vi "485 comm Main Page.vi"(8 "error in (no error)":errorcluster, 11 "Node Ptr":T3 format="%.0x") -> (0 "error out":errorcluster)   [LabVIEW 2015, in "485 comm Custom Device.lvlib"]
uses:
  485 comm Custom Device.lvlib
  <vilib>/NI Veristand/Custom Device API/Custom Device API.lvlib
  <vilib>/NI Veristand/Custom Device API/Set Item Property (U32).vi
  Serial - Settings.ctl
  <vilib>/NI Veristand/Custom Device API/Set Item Property (Boolean).vi
  <vilib>/NI Veristand/Custom Device API/Set Item Property (Variant).vi
  <vilib>/NI Veristand/Custom Device API/Get Item Property (Boolean).vi
  <vilib>/NI Veristand/Custom Device API/Set Item Property (String).vi
  <vilib>/NI Veristand/Custom Device API/Set Item Property (U16).vi
  <vilib>/NI Veristand/Custom Device API/Get Item Property (U32).vi
  <vilib>/NI Veristand/Custom Device API/Get Item Property (Variant).vi
  <vilib>/NI Veristand/Custom Device API/Get Item Property (String).vi
  <vilib>/NI Veristand/Custom Device API/Get Item Property (U16).vi
  <vilib>/NI Veristand/Custom Device API/Custom Device Channel Type.ctl
  <vilib>/NI Veristand/Custom Device API/Custom Device Channel.ctl
  <vilib>/NI Veristand/Custom Device API/Custom Device Item Ref.ctl
panel:
  in  "add output channel":bool
  in  "add input channel":bool
  in  "Reuse Old Data?":bool
  in  "Period (ms)":u32=1000
  in  "Timeout (s)":u32=10
  in  "RS-485 Transceiver Mode":T1(ring)
  in  "VISA resource":refnum<visa-resource-name>="COM3"
  in  "Serial Settings":T2={"baud rate"=9600, "data bits"=8, "parity"=enum."None", "stop bits"=10, "flow control"=0} {"flow control" items=["None"=0, "XON/XOFF"=1, "RTS/CTS"=2, "DTR/DSR"=4]; "stop bits" items=["1.0"=10, "1.5"=15, "2.0"=20]; "data bits" min=5 max=8 step=1; "baud rate" items=["75"=75, "110"=110, "134"=134, "150"=150, "300"=300, "600"=600, "1200"=1200, "1800"=1800, "2400"=2400, "4800"=4800, "7200"=7200, "9600"=9600, "14400"=14400, "19200"=19200, "28800"=28800, "38400"=38400, "56000"=56000, "57600"=57600, "115200"=115200, "128000"=128000, "230400"=230400, "921600"=921600]}
  in  "Header":cluster{"Section Name":string}={"Section Name"="Custom Device Item Settings"}
  in  "Description":string
  in  "Name":string
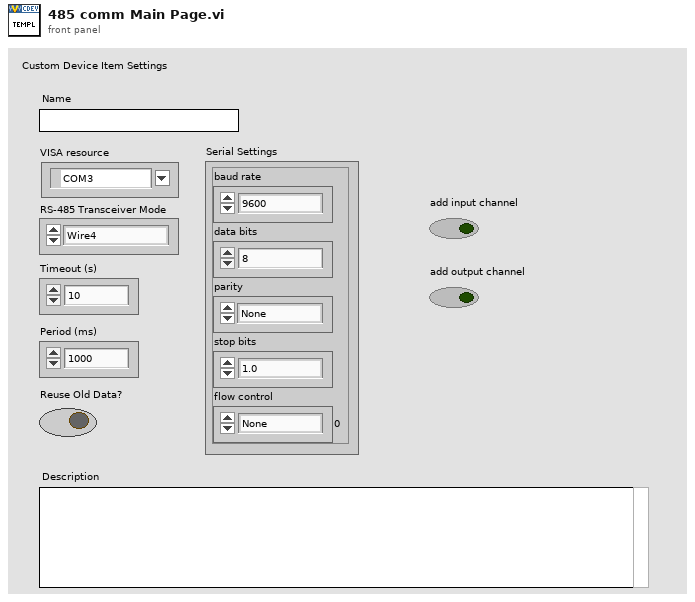
[diagram p1: front panel]
types:
  T1 = enum16{"Wire4", "Wire2-EchoDTR", "Wire2-CtrlDTR", "Wire2-Auto"}
  T2 = typedef "485 comm Custom Device.lvlib/Serial - Settings.ctl" = cluster{"baud rate":u32, "data bits":u16, "parity":enum16{"None", "Odd", "Even", "Mark", "Space"}, "stop bits":u16, "flow control":u16}
  T3 = typedef "Custom Device API.lvlib/Custom Device Item Ref.ctl" = u64
  T4 = typedef "Custom Device API.lvlib/Custom Device Item Info.ctl" = cluster{"Name":string, "Is Channel":bool, "GUID":string, "Is Waveform":bool}
  T5 = typedef "Custom Device API.lvlib/Custom Device Channel.ctl" = cluster{"Type":T6, "Units":string, "Default Value":dbl, "Faultable":bool, "Scalable":bool}
  T6 = typedef "Custom Device API.lvlib/Custom Device Channel Type.ctl" = enum16{"Input", "Output"}
  T7 = typedef "Custom Device API.lvlib/Custom Device Commands.ctl" = enum16{"Default", "Item renamed", "Shutdown", "Dynamic button pressed"}
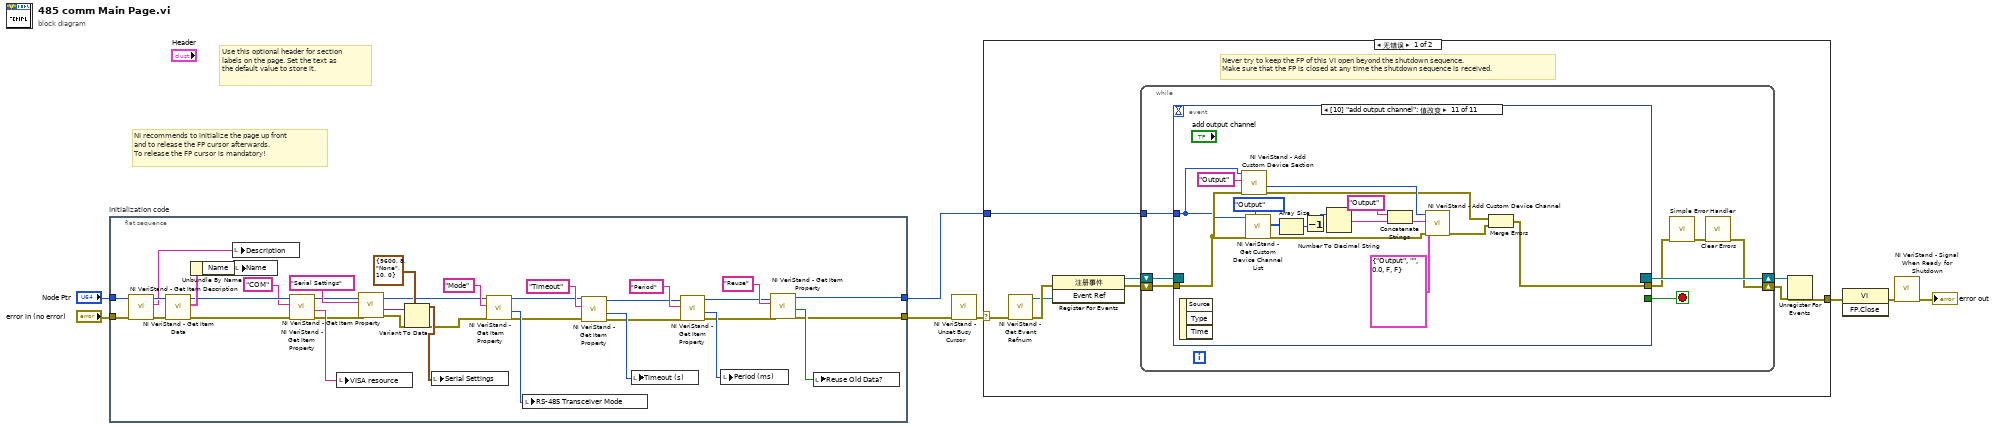
[diagram p0: block diagram]
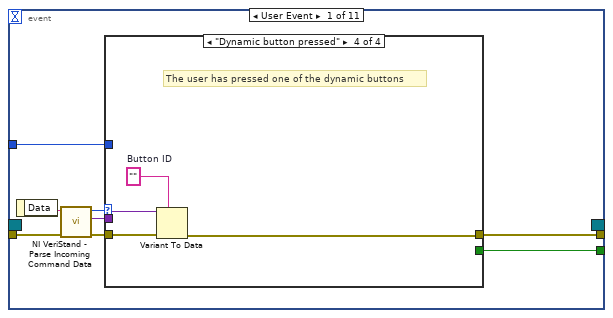
[diagram p2: hidden frame]
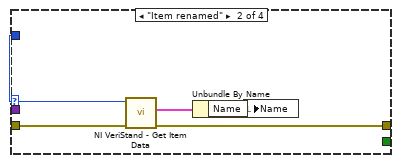
[diagram p4: hidden frame]
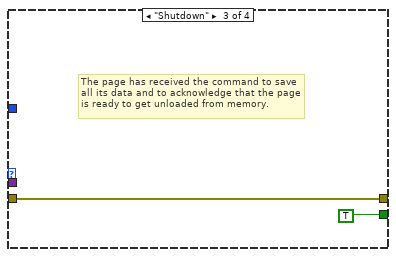
[diagram p5: hidden frame]
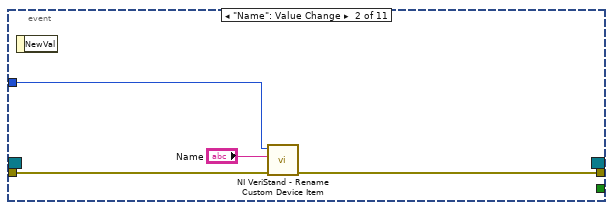
[diagram p6: hidden frame]
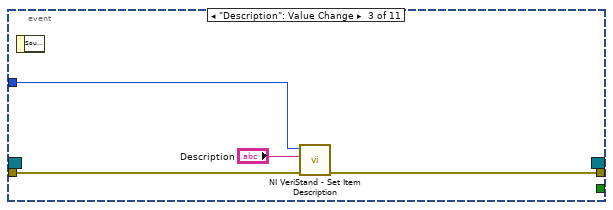
[diagram p7: hidden frame]
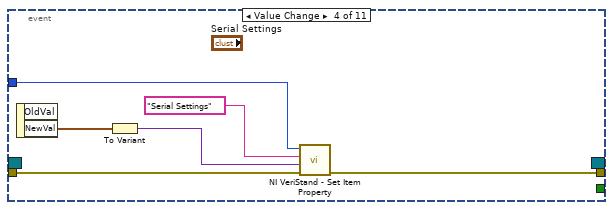
[diagram p8: hidden frame]
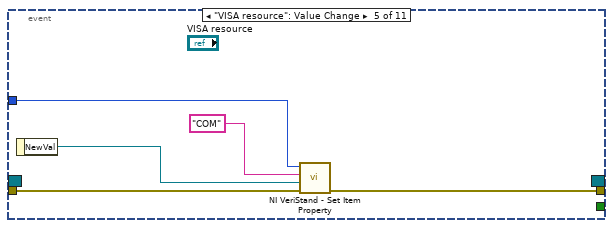
[diagram p9: hidden frame]
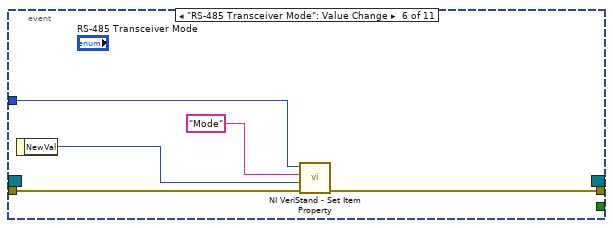
[diagram p10: hidden frame]
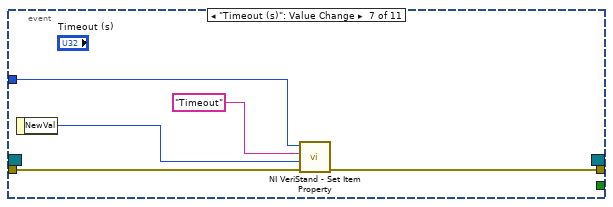
[diagram p11: hidden frame]
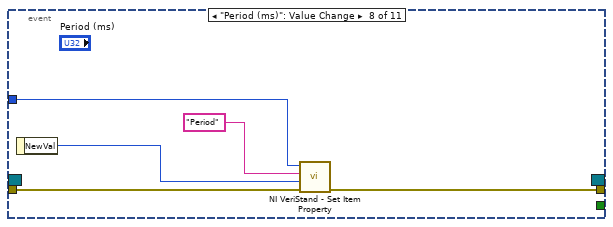
[diagram p12: hidden frame]
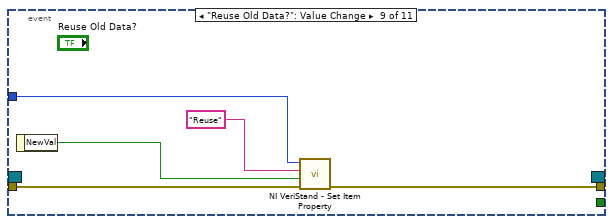
[diagram p13: hidden frame]
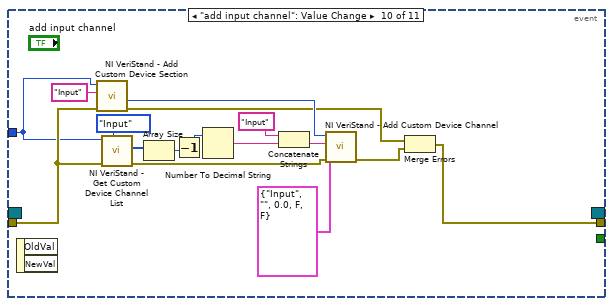
[diagram p14: hidden frame]
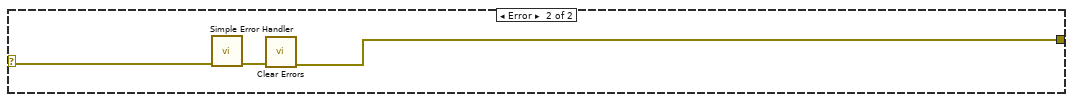
[diagram p15: hidden frame]
diagram:
  # "Use this optional header for section labels on the page. Set the text as the default value to store it."
  # "NI recommends to initialize the page up front\nand to release the FP cursor afterwards.\nTo release the FP cursor is mandatory!"
  n1 = flat-sequence "Initialization code" {
    tunnel: "error in (no error)" -> [w43]
    tunnel: "Node Ptr" -> [w42]
    tunnel: [w28] -> w4
    tunnel: [w29] -> w1
    frame #0 {
      n2 = call <vilib>:"NI VeriStand - Get Item Description.vi"("error in (no error)"=w43, "Item Ref in"=w42) -> ("error out"=w40:errorcluster, "Description"=w41:string, "Item Ref out"=w44:T3)  [unwired: 7 out]
      n3 = call <vilib>:"NI VeriStand - Get Item Data.vi"("error in (no error)"=w40, "Item Ref in"=w44) -> ("error out"=w36:errorcluster, "Item Info"=w39:T4, "Item Ref out"=w37:T3)  [unwired: 7 out]
      n4 = Unbundle By Name(w39) -> ("Name"=w38:string)
      n5 = local write "Description"(w41) -> ()
      n6 = local write "Name"(w38) -> ()
      n7 = call-poly <vilib>:"NI VeriStand - Get Item Property.vi"("error in (no error)"=w36, "Property Name"="COM", "Item Ref in"=w37) -> ("error out"=w24:errorcluster, "Value"=w34:string, "Item Ref out"=w32:T3)  [unwired: 5 in, 1 out]
      n8 = local write "VISA resource"(w34) -> ()
      n9 = call-poly <vilib>:"NI VeriStand - Get Item Property.vi"("error in (no error)"=w24, "Property Name"="Serial Settings", "Item Ref in"=w32) -> ("error out"=w23:errorcluster, "Value"=w27:variant, "Item Ref out"=w10:T3)  [unwired: 5 in, 1 out]
      n10 = Variant To Data(error in=w23, type=T2 {"baud rate"=9600, "data bits"=8, "parity"=enum."None", "stop bits"=10, "flow control"=0} ("Serial Settings 2"), Variant=w27) -> (data=w25:T2, error out=w9:errorcluster)
      n11 = local write "Serial Settings"(w25) -> ()
      n12 = call-poly <vilib>:"NI VeriStand - Get Item Property.vi"("error in (no error)"=w9, "Property Name"="Mode", "Item Ref in"=w10) -> ("error out"=w12:errorcluster, "Value"=w13:u16, "Item Ref out"=w11:T3)  [unwired: 5 in, 1 out]
      n13 = local write "RS-485 Transceiver Mode"(w13) -> ()
      n14 = call-poly <vilib>:"NI VeriStand - Get Item Property.vi"("error in (no error)"=w12, "Property Name"="Timeout", "Item Ref in"=w11) -> ("error out"=w16:errorcluster, "Value"=w18:u32, "Item Ref out"=w15:T3)  [unwired: 5 in, 1 out]
      n15 = local write "Timeout (s)"(w18) -> ()
      n16 = call-poly <vilib>:"NI VeriStand - Get Item Property.vi"("error in (no error)"=w16, "Property Name"="Period", "Item Ref in"=w15) -> ("error out"=w20:errorcluster, "Value"=w21:u32, "Item Ref out"=w19:T3)  [unwired: 5 in, 1 out]
      n17 = local write "Period (ms)"(w21) -> ()
      n18 = call-poly <vilib>:"NI VeriStand - Get Item Property.vi"("error in (no error)"=w20, "Property Name"="Reuse", "Item Ref in"=w19) -> ("error out"=w28:errorcluster, "Value"=w30:bool, "Item Ref out"=w29:T3)  [unwired: 5 in, 1 out]
      n19 = local write "Reuse Old Data?"(w30) -> ()
    }
  }
  n20 = call <vilib>:"NI VeriStand - Unset Busy Cursor.vi"("error in (no error)"=w4) -> ("error out"=w3:errorcluster)  [unwired: 10 out]
  n21 = case shown="无错误" w3 {
    selector: w3 -> [w45 w155]
    tunnel: [w50 w153] -> w8
    tunnel: w1 -> [w46 _]
    frame No Error {
      # "Never try to keep the FP of this VI open beyond the shutdown sequence.\nMake sure that the FP is closed at any time the shutdown sequence is received."
      n22 = call <vilib>:"NI VeriStand - Get Event Refnum.vi"("error in (no error)"=w45) -> ("error out"=w53:errorcluster, "Event Ref"=w49:refnum<user-event>)  [unwired: 9 out]
      n23 = register-events(error in=w53, w49) -> (reference out=w47:refnum<event-registration>, error out=w48:errorcluster)  [unwired: 1 in]
      n24 = while {
        tunnel: w46 -> [w57]
        shift-right: [w54] -> w51
        shift-left: w48 -> [w60]
        shift-right: [w61] -> w52
        shift-left: w47 -> [w59]
        stop <- w58 stop-if-true
        n25 = event shown="[10] \"add output channel\": 值改变" {
          selector: w59 -> [_ _ _ _ _ _ _ _ _ _ _]
          dyn-events: [_ _ _ _ _ _ _ _ _ _ _] -> w61
          timeout: _ -> [_ _ _ _ _ _ _ _ _ _ _]
          tunnel: w60 -> [w69 w85 w88 w94 w99 w104 w109 w114 w119 w135 w138]
          tunnel: [w65 _ _ _ _ _ _ _ _ _ _] -> w58
          tunnel: [w64 w84 w87 w93 w98 w103 w108 w113 w118 w123 w139] -> w56
          tunnel: w57 -> [w63 w83 w89 w95 w100 w105 w110 w115 w120 w134 w137]
          event User Event {
            n26 = event-data() -> ("Data"=w68:string)  [unwired: 1 out]
            n27 = call <vilib>:"NI VeriStand - Parse Incoming Command Data.vi"("error in (no error)"=w69, "Incoming data"=w68) -> ("error out"=w67:errorcluster, "Outgoing data"=w62:variant, "Action"=w66:T7)  [unwired: 7 out]
            n28 = case shown="\"Dynamic button pressed\"" w66 {
              tunnel: w67 -> [w70 w75 w76 w81]
              tunnel: [_ _ TRUE _] -> w65
              tunnel: [w70 w72 w76 w78] -> w64
              tunnel: w63 -> [_ w74 _ _]
              tunnel: w62 -> [_ _ _ w80]
              frame "Default", Default {
              }
              frame "Item renamed" {
                n29 = call <vilib>:"NI VeriStand - Get Item Data.vi"("error in (no error)"=w75, "Item Ref in"=w74) -> ("error out"=w72:errorcluster, "Item Info"=w73:T4)  [unwired: 8 out]
                n30 = Unbundle By Name(w73) -> ("Name"=w71:string)
                n31 = local write "Name"(w71) -> ()
              }
              frame "Shutdown" {
                # "The page has received the command to save all its data and to acknowledge that the page is ready to get unloaded from memory."
              }
              frame "Dynamic button pressed" {
                w79 = ""  # Button ID
                # "The user has pressed one of the dynamic buttons"
                n32 = Variant To Data(error in=w81, type=w79, Variant=w80) -> (error out=w78:errorcluster)  [unwired: 1 out]
              }
            }
          }
          event "Name": Value Change {
            n33 = event-data() -> ()  [unwired: 2 out]
            n34 = call <vilib>:"NI VeriStand - Rename Custom Device Item.vi"("error in (no error)"=w85, "New Name"="Name", "Item Ref in"=w83) -> ("error out"=w84:errorcluster)  [unwired: 1 in, 7 out]
          }
          event "Description": Value Change {
            n35 = event-data() -> ()  [unwired: 2 out]
            n36 = call <vilib>:"NI VeriStand - Set Item Description.vi"("error in (no error)"=w88, "Description"="Description", "Item Ref in"=w89) -> ("error out"=w87:errorcluster)  [unwired: 8 out]
          }
          event Value Change {
            n37 = event-data() -> ("NewVal"=w92:T2)  [unwired: 2 out]
            n38 = To Variant(anything=w92) -> (Variant=w91:variant)
            n39 = call-poly <vilib>:"NI VeriStand - Set Item Property.vi"("error in (no error)"=w94, "Value"=w91, "Property Name"="Serial Settings", "Item Ref in"=w95) -> ("error out"=w93:errorcluster)  [unwired: 5 in, 2 out]
          }
          event "VISA resource": Value Change {
            n40 = event-data() -> ("NewVal"=w96:refnum<visa-resource-name>)  [unwired: 1 out]
            n41 = call-poly <vilib>:"NI VeriStand - Set Item Property.vi"("error in (no error)"=w99, "Value"=w96, "Property Name"="COM", "Item Ref in"=w100) -> ("error out"=w98:errorcluster)  [unwired: 5 in, 2 out]
          }
          event "RS-485 Transceiver Mode": Value Change {
            n42 = event-data() -> ("NewVal"=w101:T1)  [unwired: 1 out]
            n43 = call-poly <vilib>:"NI VeriStand - Set Item Property.vi"("error in (no error)"=w104, "Value"=w101, "Property Name"="Mode", "Item Ref in"=w105) -> ("error out"=w103:errorcluster)  [unwired: 5 in, 2 out]
          }
          event "Timeout (s)": Value Change {
            n44 = event-data() -> ("NewVal"=w106:u32)  [unwired: 1 out]
            n45 = call-poly <vilib>:"NI VeriStand - Set Item Property.vi"("error in (no error)"=w109, "Value"=w106, "Property Name"="Timeout", "Item Ref in"=w110) -> ("error out"=w108:errorcluster)  [unwired: 5 in, 2 out]
          }
          event "Period (ms)": Value Change {
            n46 = event-data() -> ("NewVal"=w111:u32)  [unwired: 1 out]
            n47 = call-poly <vilib>:"NI VeriStand - Set Item Property.vi"("error in (no error)"=w114, "Value"=w111, "Property Name"="Period", "Item Ref in"=w115) -> ("error out"=w113:errorcluster)  [unwired: 5 in, 2 out]
          }
          event "Reuse Old Data?": Value Change {
            n48 = event-data() -> ("NewVal"=w116:bool)  [unwired: 1 out]
            n49 = call-poly <vilib>:"NI VeriStand - Set Item Property.vi"("error in (no error)"=w119, "Value"=w116, "Property Name"="Reuse", "Item Ref in"=w120) -> ("error out"=w118:errorcluster)  [unwired: 5 in, 2 out]
          }
          event "add input channel": Value Change {
            n50 = event-data() -> ()  [unwired: 3 out]
            n51 = call <vilib>:"NI VeriStand - Add Custom Device Section.vi"("error in (no error)"=w135, "Section Name"="Input", "Parent Ref in"=w134) -> ("error out"=w124:errorcluster, "Section Ptr"=w131:T3)  [unwired: 5 in, 2 out]
            n52 = call <vilib>:"NI VeriStand - Get Custom Device Channel List.vi"("Channel Type"=Custom_Device_Channel_Type."Input", "error in (no error)"=w135, "Device Ref in"=w134) -> ("error out"=w132:errorcluster, "Specified Channel Ref List"=w136:T3[])  [unwired: 6 in, 1 out]
            n53 = Array Size(array=w136) -> (size(s)=w129:i32)
            n54 = Decrement(x=w129) -> (x-1=w128:i32)
            n55 = Number To Decimal String(number=w128) -> (decimal integer string=w127:string)  [unwired: 1 in]
            n56 = Concatenate Strings("Input" ("字符串"), w127) -> (w130:string)
            n57 = call <vilib>:"NI VeriStand - Add Custom Device Channel.vi"("error in (no error)"=w132, "Channel"=T5 {"Type"=enum."Input", "Units"="", "Default Value"=0.0, "Faultable"=FALSE, "Scalable"=FALSE}, "Channel Name"=w130, "Parent Ref in"=w131) -> ("error out"=w125:errorcluster)  [unwired: 4 in, 3 out]
            n58 = Merge Errors(w124, w125) -> (w123:errorcluster)
          }
          event "add output channel": Value Change {
            n59 = event-data() -> ()  [unwired: 4 out]
            n60 = call <vilib>:"NI VeriStand - Add Custom Device Section.vi"("error in (no error)"=w138, "Section Name"="Output", "Parent Ref in"=w137) -> ("error out"=w142:errorcluster, "Section Ptr"=w149:T3)  [unwired: 5 in, 2 out]
            n61 = call <vilib>:"NI VeriStand - Get Custom Device Channel List.vi"("Channel Type"=Custom_Device_Channel_Type."Output", "error in (no error)"=w138, "Device Ref in"=w137) -> ("error out"=w150:errorcluster, "Specified Channel Ref List"=w152:T3[])  [unwired: 6 in, 1 out]
            n62 = Array Size(array=w152) -> (size(s)=w147:i32)
            n63 = Decrement(x=w147) -> (x-1=w146:i32)
            n64 = Number To Decimal String(number=w146) -> (decimal integer string=w145:string)  [unwired: 1 in]
            n65 = Concatenate Strings("Output" ("字符串"), w145) -> (w148:string)
            n66 = call <vilib>:"NI VeriStand - Add Custom Device Channel.vi"("error in (no error)"=w150, "Channel"=T5 {"Type"=enum."Output", "Units"="", "Default Value"=0.0, "Faultable"=FALSE, "Scalable"=FALSE}, "Channel Name"=w148, "Parent Ref in"=w149) -> ("error out"=w143:errorcluster)  [unwired: 4 in, 3 out]
            n67 = Merge Errors(w142, w143) -> (w139:errorcluster)
          }
        }
        n68 = call <vilib>:"Simple Error Handler.vi"("error in (no error)"=w56) -> ("error out"=w55:errorcluster)  [unwired: 1 in, 7 out]
        n69 = call <vilib>:"Clear Errors.vi"("error in (no error)"=w55) -> ("error out"=w54:errorcluster)  [unwired: 1 in, 5 out]
      }
      n70 = Unregister For Events(event registration refnum=w52, error in=w51) -> (error out=w50:errorcluster)
    }
    frame Error {
      n71 = call <vilib>:"Simple Error Handler.vi"("error in (no error)"=w155) -> ("error out"=w154:errorcluster)  [unwired: 1 in, 7 out]
      n72 = call <vilib>:"Clear Errors.vi"("error in (no error)"=w154) -> ("error out"=w153:errorcluster)  [unwired: 1 in, 5 out]
    }
  }
  n73 = invoke class="VI" method="FP.Close"(error in=w8) -> (error out=w7:errorcluster)  [unwired: 2 in, 2 out]
  n74 = call <vilib>:"NI VeriStand - Signal When Ready for Shutdown.vi"("error in (no error)"=w7) -> ("error out"=→"error out":errorcluster)  [unwired: 10 out]
